vi "iniDrivers.vi"(6 "INI Options":T1, 7 "Section":string, 8 "Error In":errorcluster, 9 "Value":string, 10 "Key":string, 11 "File Path In":path) -> (0 "Error Out":errorcluster, 2 "Value Out":string[][](array[string]), 3 "File Path Out":path)   [LabVIEW 2018]
uses:
  controls/iniDriverSelectorEnum.ctl
  <vilib>/Utility/config.llb/Write Key (String).vi
  <vilib>/Utility/config.llb/Read Key (String).vi
  <vilib>/Utility/config.llb/NI_LVConfig.lvlib
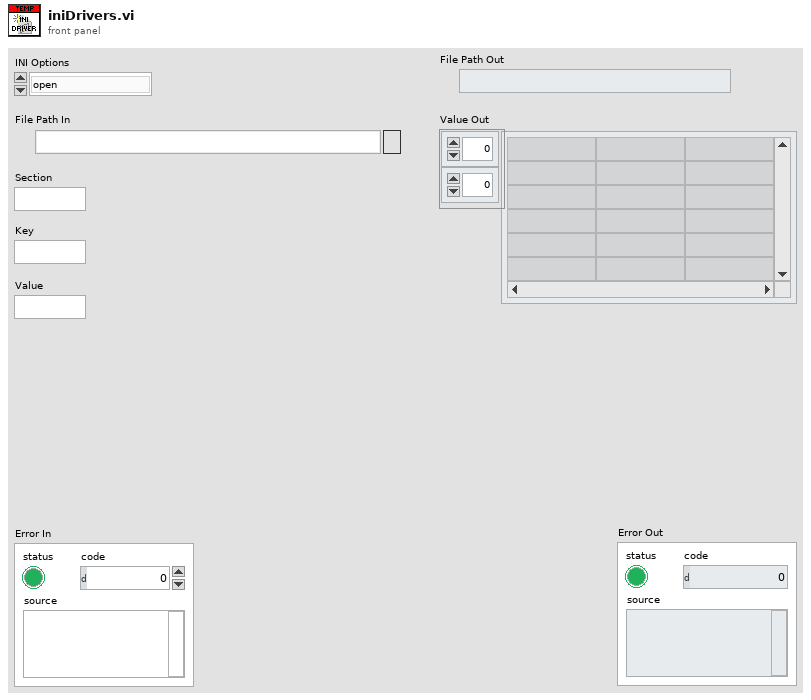
[diagram p1: front panel]
types:
  T1 = typedef "iniDriverSelectorEnum.ctl" = enum16{"open", "Write", "Read", "close"}
  T2 = typedef "NI_LVConfig.lvlib/Config Data RefNum.ctl" = refnum<k1>
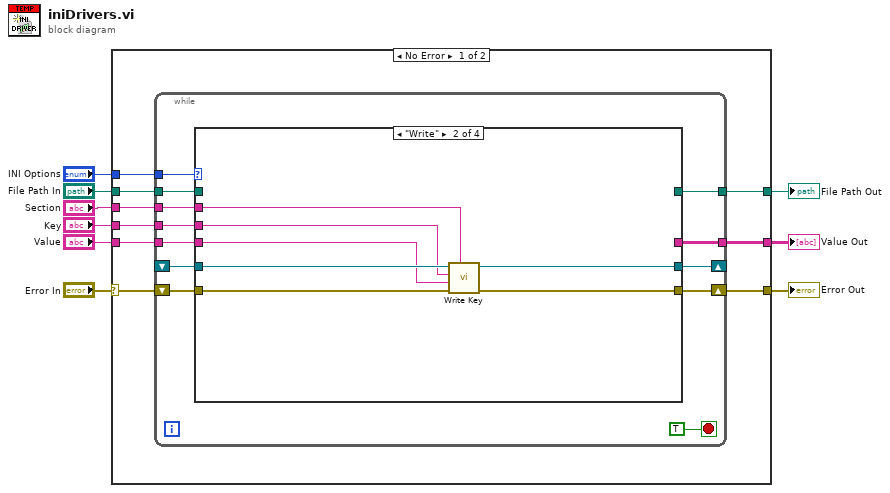
[diagram p0: block diagram]
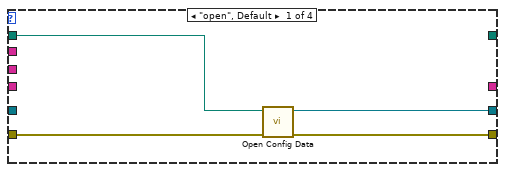
[diagram p2: hidden frame]
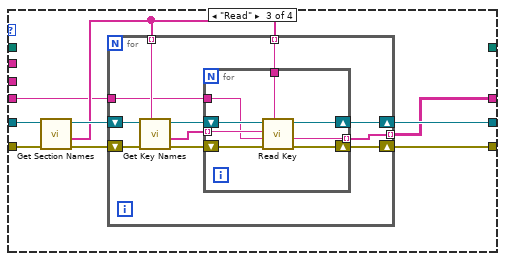
[diagram p3: hidden frame]
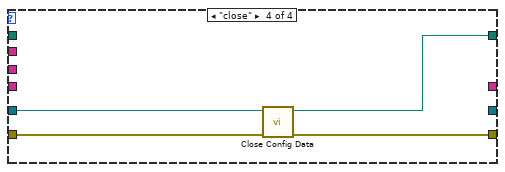
[diagram p4: hidden frame]
diagram:
  n1 = case shown="No Error" "Error In" {
    selector: "Error In" -> [w18 w74]
    tunnel: [w17 w74] -> w8
    tunnel: "INI Options" -> [w16 _]
    tunnel: "File Path In" -> [w15 _]
    tunnel: "Section" -> [w14 _]
    tunnel: "Key" -> [w13 _]
    tunnel: "Value" -> [w12 _]
    tunnel: [w11 _] -> w2
    tunnel: [w10 _] -> w1
    frame No Error {
      n2 = while {
        tunnel: w16 -> [w28]
        shift-right: [w29] -> w17
        shift-left: w18 -> [w30]
        shift-right: [w27] -> _
        shift-left: _ -> [w26]
        tunnel: w15 -> [w25]
        tunnel: w14 -> [w24]
        tunnel: w13 -> [w23]
        tunnel: w12 -> [w22]
        tunnel: [w21] -> w11
        tunnel: [w20] -> w10
        stop <- TRUE stop-if-true
        n3 = case shown="\"Write\"" w28 {
          tunnel: w30 -> [w33 w40 w47 w71]
          tunnel: [w34 w41 w50 w73] -> w29
          tunnel: [w32 w39 w49 _] -> w27
          tunnel: w26 -> [_ w38 w48 w72]
          tunnel: w25 -> [w31 _ _ _]
          tunnel: w24 -> [_ w37 _ _]
          tunnel: w23 -> [_ w36 _ _]
          tunnel: w22 -> [_ w35 w42 _]
          tunnel: [_ _ w43 _] -> w21
          tunnel: [_ _ _ w70] -> w20
          frame "open", Default {
            n4 = call <vilib>:"Open Config Data.vi"("error in (no error)"=w33, "configuration file path"=w31) -> ("error out"=w34:errorcluster, "refnum"=w32:T2)  [unwired: 7 in, 1 out]
          }
          frame "Write" {
            n5 = call-poly <vilib>:"Write Key.vi"("section"=w37, "error in (no error)"=w40, "value"=w35, "key"=w36, "refnum"=w38) -> ("error out"=w41:errorcluster, "refnum out"=w39:T2)  [unwired: 4 in, 1 out]
          }
          frame "Read" {
            n6 = call <vilib>:"Get Section Names.vi"("error in (no error)"=w47, "refnum"=w48) -> ("error out"=w45:errorcluster, "section names"=w44:string[], "refnum out"=w46:T2)  [unwired: 7 in]
            n7 = for {
              shift-right: [w60] -> w49
              shift-left: w46 -> [w57]
              shift-right: [w61] -> w50
              shift-left: w45 -> [w58]
              tunnel: w44 -> [w59] mode=indexing
              tunnel: w44 -> [w54] mode=indexing
              tunnel: [w52] -> w43 mode=indexing
              tunnel: w42 -> [w51]
              n8 = call <vilib>:"Get Key Names.vi"("section"=w54, "error in (no error)"=w58, "refnum"=w57) -> ("error out"=w55:errorcluster, "key names"=w53:string[], "refnum out"=w56:T2)  [unwired: 5 in, 1 out]
              n9 = for {
                tunnel: w59 -> [w67]
                shift-right: [w68] -> w60
                shift-left: w56 -> [w66]
                shift-right: [w69] -> w61
                shift-left: w55 -> [w65]
                tunnel: w53 -> [w64] mode=indexing
                tunnel: [w63] -> w52 mode=indexing
                tunnel: w51 -> [w62]
                n10 = call-poly <vilib>:"Read Key.vi"("section"=w67, "error in (no error)"=w65, "default value"=w62, "key"=w64, "refnum"=w66) -> ("error out"=w69:errorcluster, "value"=w63:string, "refnum out"=w68:T2)  [unwired: 3 in, 1 out]
              }
            }
          }
          frame "close" {
            n11 = call <vilib>:"Close Config Data.vi"("error in (no error)"=w71, "refnum"=w72) -> ("error out"=w73:errorcluster, "file path"=w70:path)  [unwired: 8 in]
          }
        }
      }
    }
    frame Error {
    }
  }
  "Error Out" <- w8
  "Value Out" <- w2
  "File Path Out" <- w1
